vi "S2DS_ErrorCheckingInX (unitless).vi"(0 "Scan parameters in":T1 {"Y data taking" items=["in both direction", "in up direction only", "in down direction only"]; "X data taking" items=["in both direction", "in up direction only", "in down direction only"]}) -> (1 "Error string":string, 2 "Error?":bool)   [LabVIEW 2025]
uses:
  TYPE DEFS/S2DS_Sweep Info.ctl
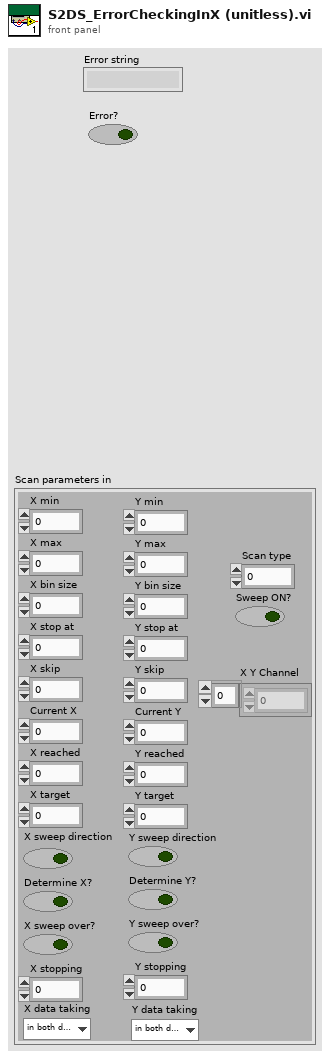
[diagram p1: front panel]
types:
  T1 = typedef "S2DS_Sweep Info.ctl" = cluster{"X min":ext, "X max":dbl, "Y min":dbl, "Y max":dbl, "X bin size":dbl, "Y bin size":dbl, "X stop at":dbl, "Y stop at":dbl, "X skip":u64, "Y skip":u64, "Current X":dbl, "Current Y":dbl, "X reached":i32, "Y reached":i32, "X target":dbl, "Y target":dbl, "Sweep ON?":bool, "X sweep direction":bool, "Y sweep direction":bool, "Determine X?":bool, "Determine Y?":bool, "X sweep over?":bool, "Y sweep over?":bool, "Scan type":i32, "X stopping":i32, "Y stopping":i32, "X Y Channel":u16[], "X data taking":u16, "Y data taking":u16}
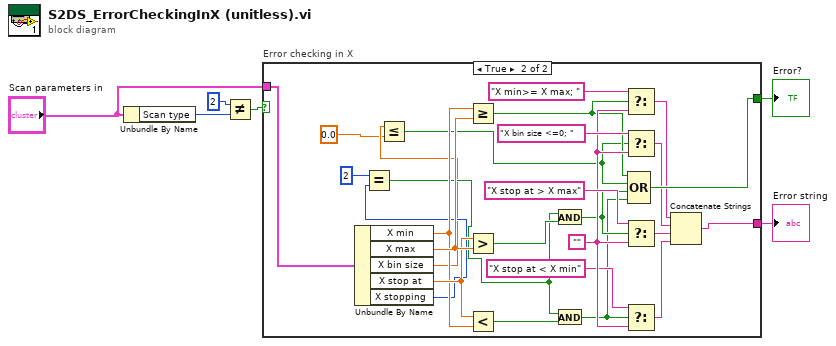
[diagram p0: block diagram]
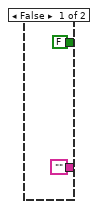
[diagram p2: hidden frame]
diagram:
  n1 = Unbundle By Name("Scan parameters in") -> ("Scan type"=w4:i32)
  n2 = Not Equal?(x=2, y=w4) -> (x != y?=w5:bool)
  n3 = case "Error checking in X" shown="True" w5 {
    tunnel: "Scan parameters in" -> [_ w34]
    tunnel: [FALSE w20] -> w1
    tunnel: ["" w15] -> w2
    frame False {
    }
    frame True {
      w25 = ""
      n4 = Unbundle By Name(w34) -> ("X min"=w27:ext, "X max"=w31:dbl, "X bin size"=w11:dbl, "X stop at"=w28:dbl, "X stopping"=w14:i32)
      n5 = Equal?(x=2, y=w14) -> (x = y?=w12:bool)
      n6 = Less Or Equal?(x=w11, y=0.0) -> (x <= y?=w9:bool)
      n7 = Greater Or Equal?(x=w27, y=w31) -> (x >= y?=w23:bool)
      n8 = Greater?(x=w28, y=w31) -> (0:w30:bool)
      n9 = Less?(x=w28, y=w27) -> (x < y?=w26:bool)
      n10 = And(x=w12, y=w30) -> (x .and. y?=w22:bool)
      n11 = And(x=w12, y=w26) -> (x .and. y?=w21:bool)
      n12 = Select(t="X min>= X max; ", s=w23, f=w25) -> (s? t:f=w19:string)
      n13 = Select(t="X bin size <=0; ", s=w9, f=w25) -> (s? t:f=w18:string)
      n14 = Select(t="X stop at > X max", s=w22, f=w25) -> (s? t:f=w17:string)
      n15 = Select(t="X stop at < X min", s=w21, f=w25) -> (s? t:f=w16:string)
      n16 = Compound Arithmetic op=OR(w23, w9, w22, w21) -> (w20:bool)
      n17 = Concatenate Strings(w19, w18, w17, w16) -> (w15:string)
    }
  }
  "Error string" <- w2
  "Error?" <- w1
